vi "KDH_EX3Task2_Main.vi"() -> ()   [LabVIEW 2014, in "Harris_MacMaster_4th_LEGORobotics_11-29-16.lvrbt"]
uses:
  Harris_MacMaster_4th_LEGORobotics_11-29-16.lvrbt
  <vilib>/NXT/Block Support/NXT_InputPort.ctl
  <vilib>/NXT/Block Support/NXT_OutputPort.ctl
  <vilib>/NXT/Dual Mode Library/Sensors/EV3_Ultrasonic_CM.vi
  <vilib>/NXT/NXTIO Xnodes/NXTIONodeSubVIs/NXTMoveMotors.vi
  <vilib>/NXT/NXTIO Xnodes/AddressXNode/NXTIOAddress.xnode
  <vilib>/NXT/Subs/LVHSConnector.ctl
  <vilib>/NXT/NXTIO Xnodes/NXTIOXNode/NXTIO.xnode
  <vilib>/NXT/LegoClasses/BrickReference/BrickReference.lvclass
panel:
  in  "stop button":bool
  out "final iteration value":i32
  out "number of loop interations":i32
  out "current iteration":i32
  out "distance from wall":dbl
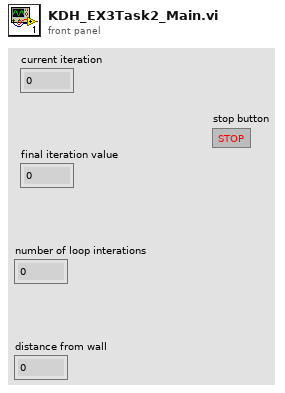
[diagram p1: front panel]
types:
  T1 = typedef "NXT_OutputPort.ctl" = u8
  T2 = typedef "NXT_InputPort.ctl" = u32
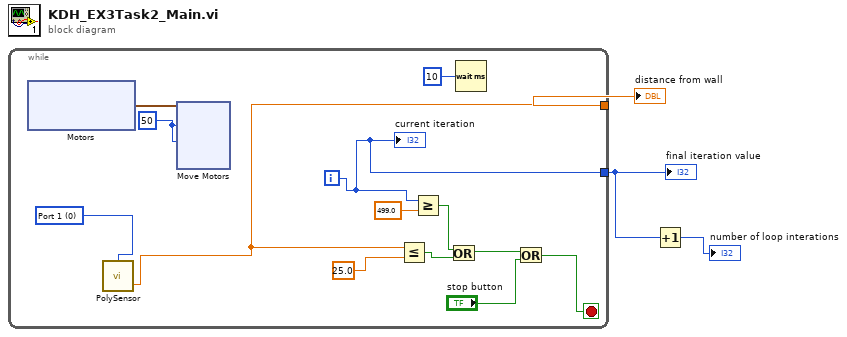
[diagram p0: block diagram]
diagram:
  n1 = while {
    tunnel: [w13] -> w3
    tunnel: [w5] -> w1
    i -> [w5]
    stop <- w7 stop-if-true
    w4 = i8 50 ("Power/Speed 1")
    w12 = T2 0 items=["Port 1", "Port 2", "Port 3", "Port 4"] ("Port (Port 1)")
    n2 = xnode "Motors"() -> ("Motor"=w15:cluster{"Port":T1, "Port":T1})
    n3 = call-poly <vilib>:"PolySensor.vi"("Port (Port 1)"=w12) -> ("Centimeters"=w13:sgl)  [unwired: 2 in, 1 out]
    n4 = xnode "Move Motors"("Power/Speed 2"=w4, "Power/Speed 1"=w4, "Motors"=w15) -> ()  [unwired: 1 in, 1 out]
    n5 = Less Or Equal?(x=w13, y=25.0) -> (x <= y?=w11:bool)
    n6 = Greater Or Equal?(x=w5, y=499.0) -> (x >= y?=w10:bool)
    n7 = Or(x=w10, y=w11) -> (x .or. y?=w8:bool)
    n8 = Wait (ms)(milliseconds to wait=u32 10) -> ()  [unwired: 1 out]
    n9 = Or(x=w8, y="stop button") -> (x .or. y?=w7:bool)
    "current iteration" <- w5
  }
  "distance from wall" <- w3
  "final iteration value" <- w1
  n10 = Increment(x=w1) -> (x+1=→"number of loop interations":i32)
